vi "GXMLTest.vi"() -> ()   [LabVIEW 2015]
uses:
  <vilib>/NI/GXML/_subVIs/GXML SearchParser/Search Parser.vi
  <vilib>/NI/GXML/GXML.lvlib
panel:
  in  "Write?":bool
  in  "XML File Path":path=path "C:/SoftwareDevelopment/Workspace_2017/XpathTest/src/xpathTest/gxmlExport.xml"
  out "Concatenated GXML String":string
  in  "PID":T1
  in  "encoder":T2
  in  "limit":T3
  in  "template":T4
  in  "motor":T5
  in  "xmlEntries":enum32{"IntakeLift", "ChooChoo"}(tab)
  in  "c":bool
  in  "a":dbl
  in  "IntakeLift":T4
  in  "E":dbl
  in  "D":dbl
  out "B":bool
  in  "ChooChoo":T4
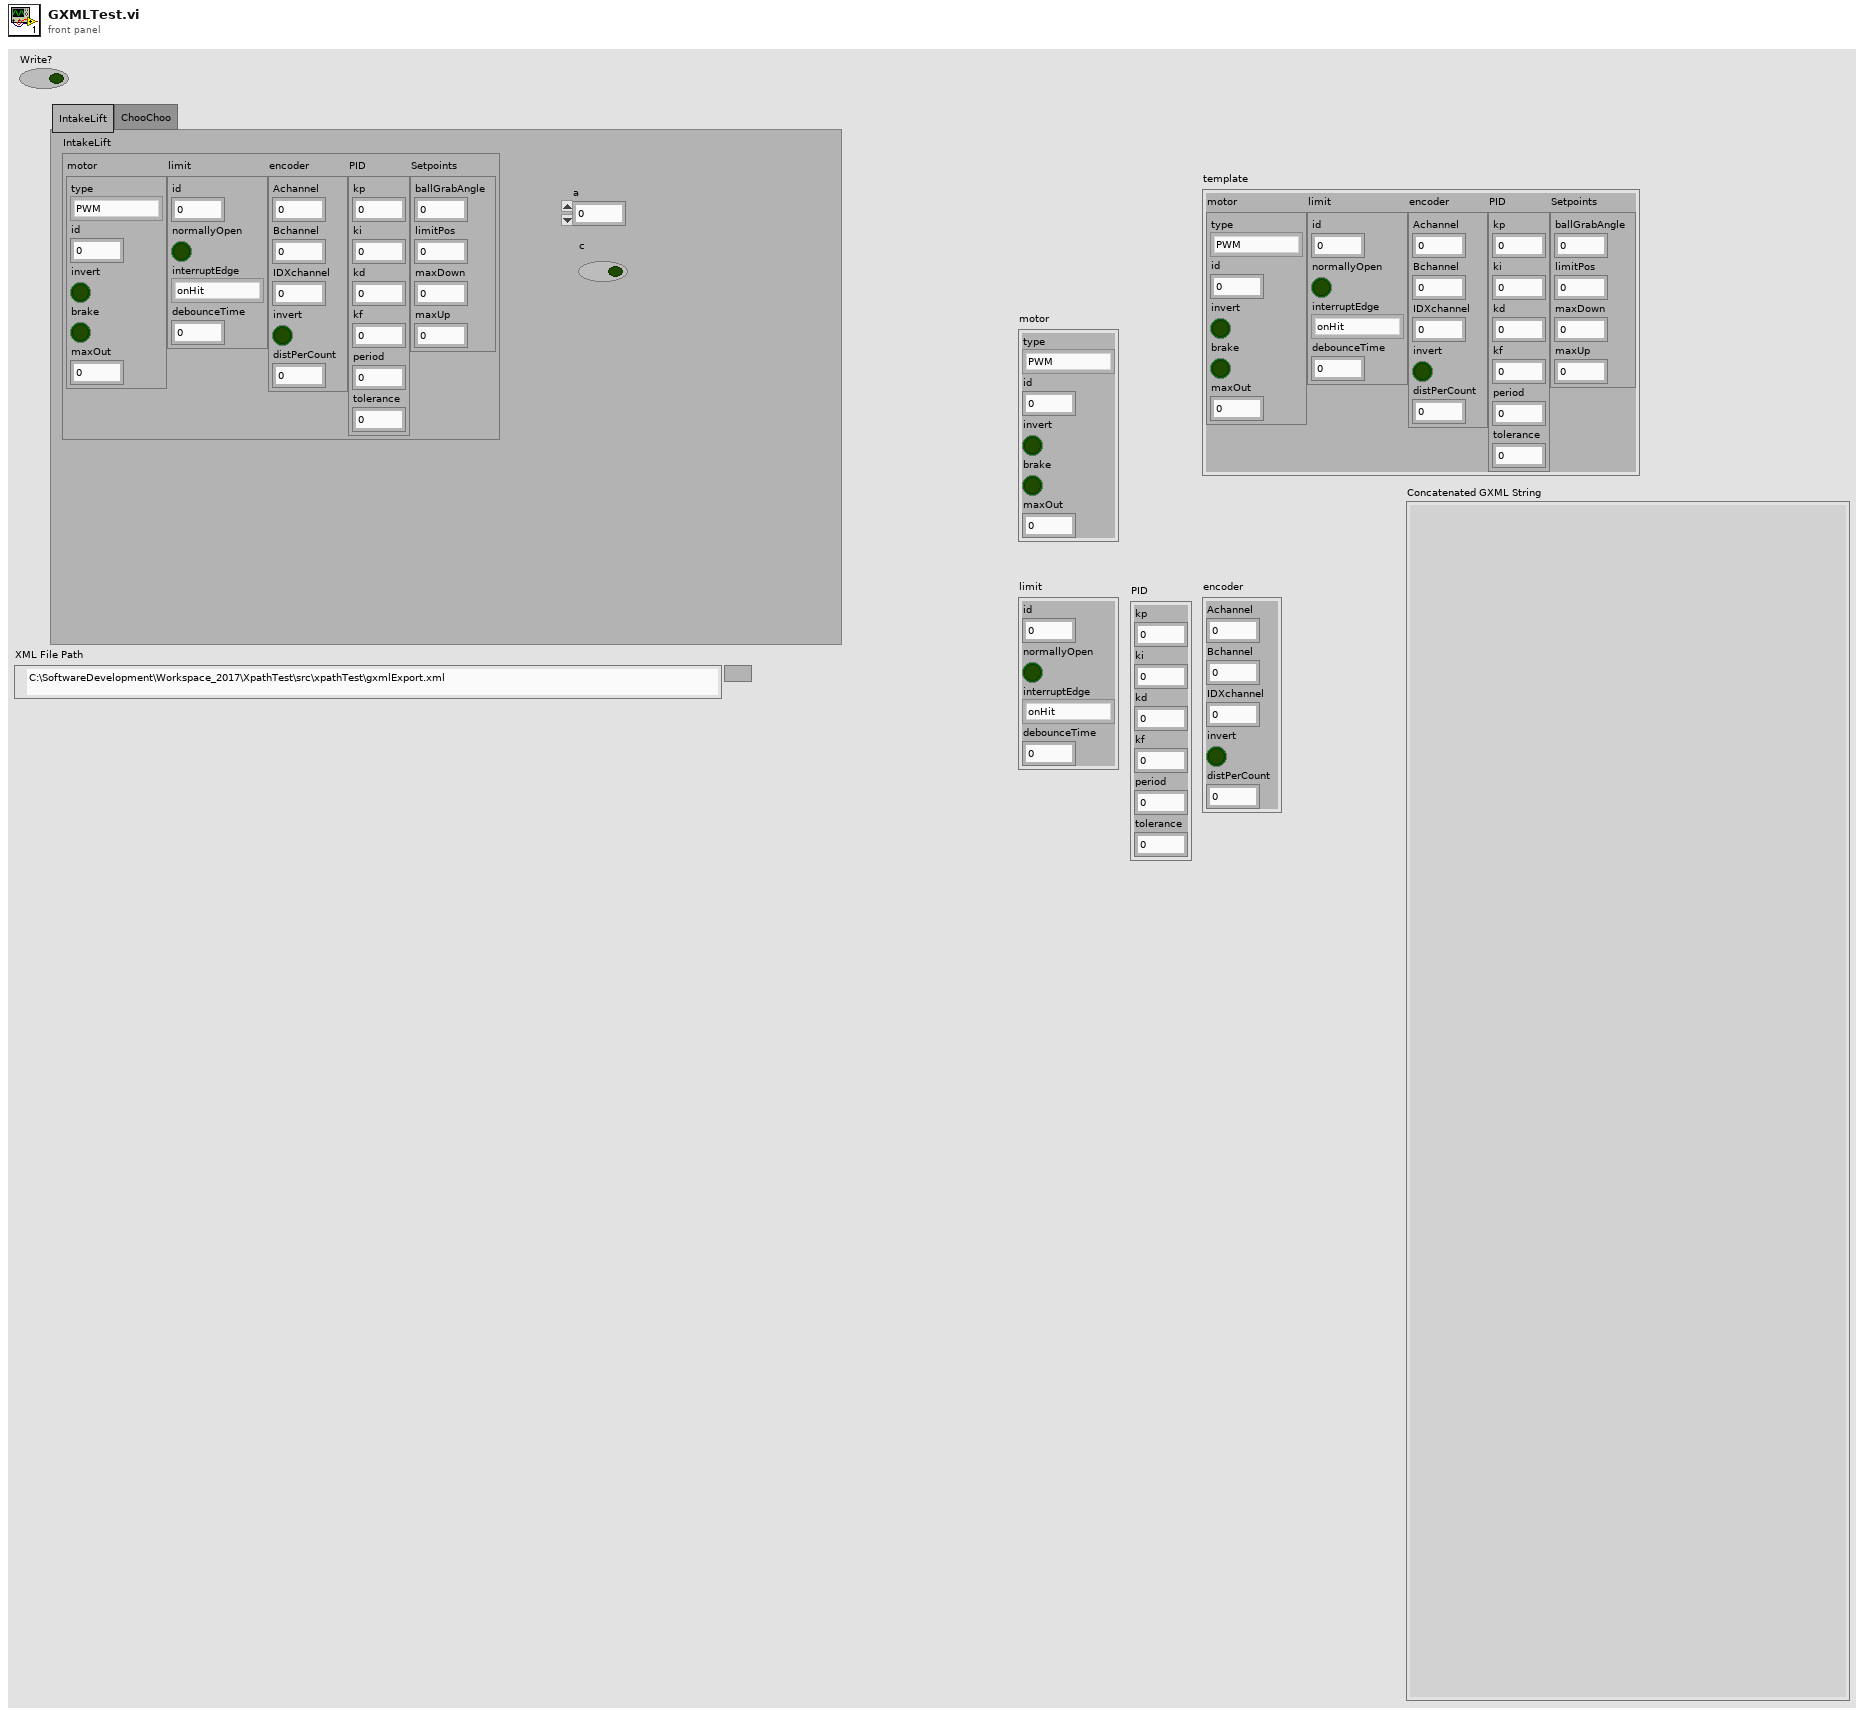
[diagram p1: front panel]
types:
  T1 = cluster{"kp":dbl, "ki":dbl, "kd":dbl, "kf":dbl, "period":dbl, "tolerance":dbl}
  T2 = cluster{"Achannel":i32, "Bchannel":i32, "IDXchannel":i32, "invert":bool, "distPerCount":dbl}
  T3 = cluster{"id":i32, "normallyOpen":bool, "interruptEdge":enum16{"onHit", "onRelease", "both"}, "debounceTime":dbl}
  T4 = cluster{"motor":cluster{"type":enum16{"PWM", "CANTalon"}, "id":i32, "invert":bool, "brake":bool, "maxOut":dbl}, "limit":cluster{"id":i32, "normallyOpen":bool, "interruptEdge":enum16{"onHit", "onRelease", "both"}, "debounceTime":dbl}, "encoder":cluster{"Achannel":i32, "Bchannel":i32, "IDXchannel":i32, "invert":bool, "distPerCount":dbl}, "PID":cluster{"kp":dbl, "ki":dbl, "kd":dbl, "kf":dbl, "period":dbl, "tolerance":dbl}, "Setpoints":cluster{"ballGrabAngle":dbl, "limitPos":dbl, "maxDown":dbl, "maxUp":dbl}}
  T5 = cluster{"type":enum16{"PWM", "CANTalon"}, "id":i32, "invert":bool, "brake":bool, "maxOut":dbl}
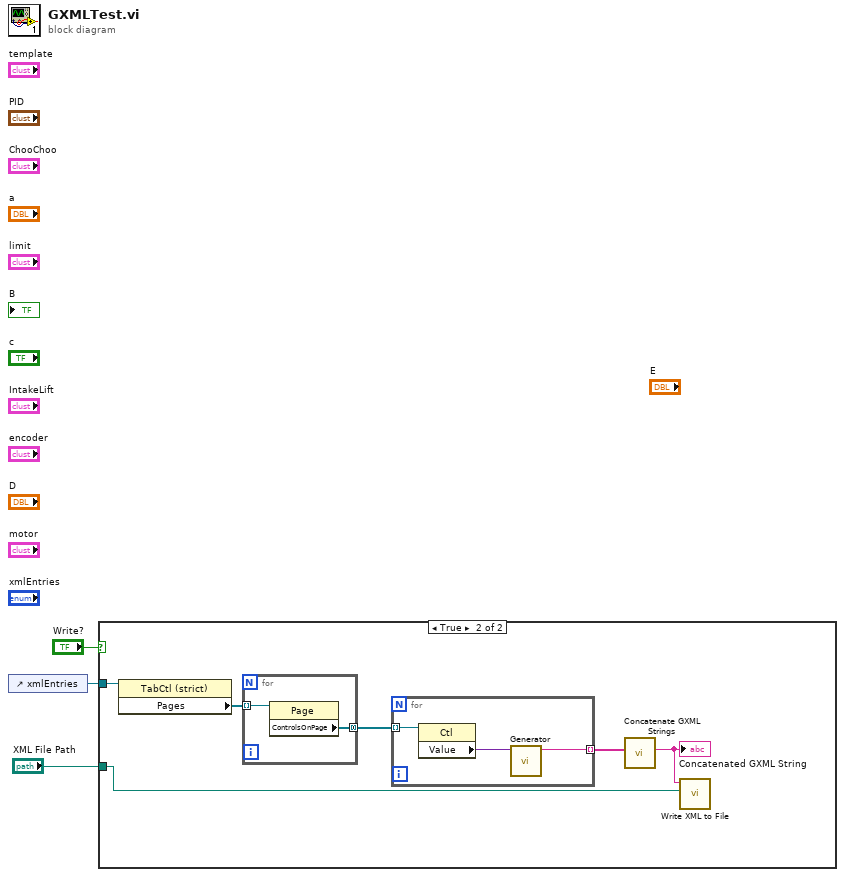
[diagram p0: block diagram]
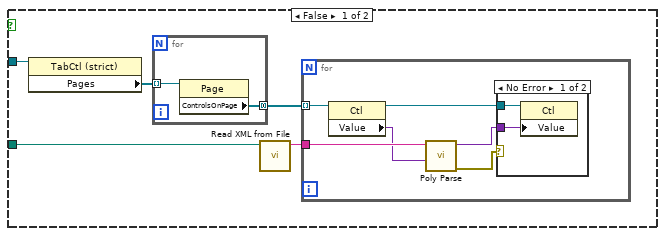
[diagram p2: hidden frame]
diagram:
  n1 = control-ref of="xmlEntries"() -> (w1:refnum<vi>)
  n2 = case shown="True" "Write?" {
    tunnel: "XML File Path" -> [w5 w20]
    tunnel: w1 -> [w6 w19]
    frame False {
      n3 = property class="TabCtl (strict)"(reference=w6) -> ("Pages"=w8:refnum<vi>[])  [unwired: 1 in, 2 out]
      n4 = for {
        tunnel: w8 -> [w18] mode=indexing
        tunnel: [w17] -> w7 mode=concatenating
        n5 = property class="Page"(reference=w18) -> ("ControlsOnPage"=w17:refnum<vi>[])  [unwired: 1 in, 2 out]
      }
      n6 = call <vilib>:"Read XML from File.vi"("XML File Path"=w5) -> ("XML String Out"=w4:string)  [unwired: 9 in, 1 out]
      n7 = for {
        tunnel: w7 -> [w14] mode=indexing
        tunnel: w4 -> [w13]
        n8 = property class="Ctl"(reference=w14) -> (reference out=w10:refnum<vi>, "Value"=w12:variant)  [unwired: 1 in, 1 out]
        n9 = call-poly <vilib>:"Poly Parse.vi"("TypeDesc"=w12, "XML String In"=w13) -> ("error out"=w9:errorcluster, "Parsed Data"=w11:variant)  [unwired: 8 in]
        n10 = case shown="No Error" w9 {
          tunnel: w11 -> [w16 _]
          tunnel: w10 -> [w15 _]
          frame No Error {
            n11 = property class="Ctl"(reference=w15, "Value"=w16) -> ()  [unwired: 1 in, 2 out]
          }
          frame Error {
          }
        }
      }
    }
    frame True {
      n12 = property class="TabCtl (strict)"(reference=w19) -> ("Pages"=w24:refnum<vi>[])  [unwired: 1 in, 2 out]
      n13 = for {
        tunnel: w24 -> [w29] mode=indexing
        tunnel: [w28] -> w23 mode=concatenating
        n14 = property class="Page"(reference=w29) -> ("ControlsOnPage"=w28:refnum<vi>[])  [unwired: 1 in, 2 out]
      }
      n15 = for {
        tunnel: w23 -> [w27] mode=indexing
        tunnel: [w25] -> w22 mode=indexing
        n16 = property class="Ctl"(reference=w27) -> ("Value"=w26:variant)  [unwired: 1 in, 2 out]
        n17 = call <vilib>:"Generator.vi"("Variant"=w26) -> ("XML String Out"=w25:string)  [unwired: 9 in, 1 out]
      }
      n18 = call <vilib>:"Concatenate GXML Strings.vi"("GXML Strings"=w22) -> ("Concatenated GXML String"=w21:string)  [unwired: 9 in, 1 out]
      "Concatenated GXML String" <- w21
      n19 = call <vilib>:"Write XML to File.vi"("XML File Path"=w20, "XML Input"=w21) -> ()  [unwired: 9 in, 1 out]
    }
  }
